vi "Tracks Button Adjust.vi"(0 "Left Forward Adjust":bool, 1 "Left Reverse Adjust":bool, 2 "Right Forward Adjust":bool, 3 "Right Reverse Adjust":bool, 4 "Adjust Speed":dbl, 5 "Drive 1":string="RobotDrive") -> ()   [LabVIEW 2017]
uses:
  <vilib>/Rock Robotics/WPI/Utilities/WPI_GetSetVariantRefNum.vi
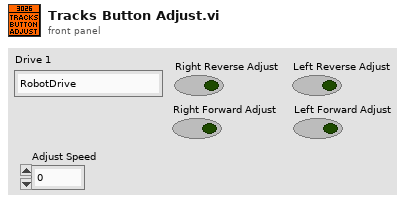
[diagram p1: front panel]
types:
  T1 = typedef "WPI_RobotDriveDevRef.ctl" = cluster{"DevStatus":errorcluster, "Motors[]":T2[], "Square Inputs":bool, "Max Output":dbl}
  T2 = typedef "WPI_MotorControlDeviceRef.ctl" = cluster{"DeviceStatus":errorcluster, "Type":T3, "PWM":cluster{"PWM Channel":T4, "DeadBand":T5}, "CAN":cluster{"Device Number":u8, "SetOutput VI Ref":variant, "GetOutput VI Ref":variant, "Enable VI Ref":variant, "Disable VI Ref":variant, "Data":variant}, "Invert":bool, "DIO PWM":cluster{"PWM \"Enable\" Channel":T4, "DIOChannel":T6, "PWM Rate":dbl}}
  T3 = typedef "WPI_MotorControlType.ctl" = enum16{"PWM", "CAN", "DIO PWM"}
  T4 = typedef "FPGA_DIOPWMChannel.ctl" = enum8{"PWM 0", "PWM 1", "PWM 2", "PWM 3", "PWM 4", "PWM 5", "PWM 6", "PWM 7", "PWM 8", "PWM 9", "PWM MXP 0", "PWM MXP 1", "PWM MXP 2", "PWM MXP 3", "PWM MXP 4", "PWM MXP 5", "PWM MXP 6", "PWM MXP 7", "PWM MXP 8", "PWM MXP 9", "Invalid"}
  T5 = typedef "WPI_PWMDeadband.ctl" = cluster{"Name":string, "maxPositivePwm":i32, "minPositivePwm":i32, "centerPwm":i32, "maxNegativePwm":i32, "minNegativePwm":i32, "angularRange":u16}
  T6 = typedef "FPGA_DIOChannel.ctl" = enum8{"DIO 0", "DIO 1", "DIO 2", "DIO 3", "DIO 4", "DIO 5", "DIO 6", "DIO 7", "DIO 8", "DIO 9", "DIO MXP 0", "DIO MXP 1", "DIO MXP 2", "DIO MXP 3", "DIO MXP 4", "DIO MXP 5", "DIO MXP 6", "DIO MXP 7", "DIO MXP 8", "DIO MXP 9", "DIO MXP 10", "DIO MXP 11", "DIO MXP 12", "DIO MXP 13", "DIO MXP 14", "DIO MXP 15", "SPI Port CS1", "SPI Port CS2", "SPI Port CS3", "SPI Port MISO", "SPI Port MOSI", "Invalid"}
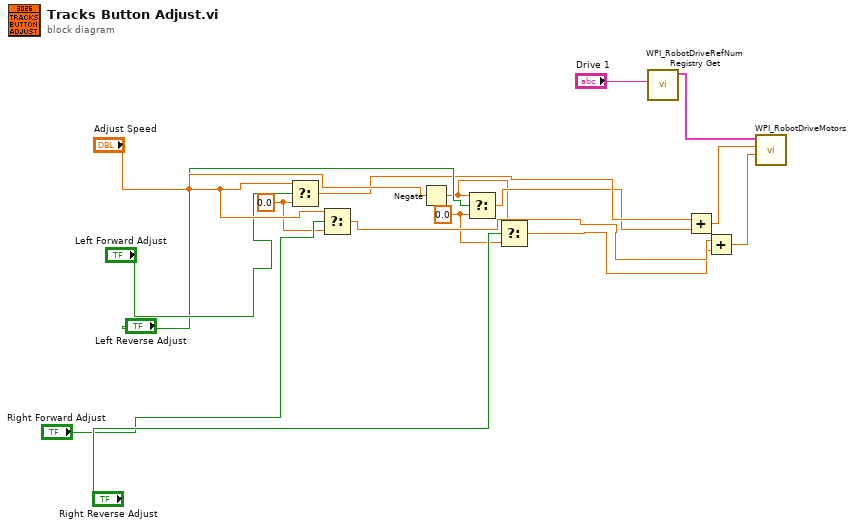
[diagram p0: block diagram]
diagram:
  w2 = 0.0 ("f")
  w1 = 0.0 ("f")
  n1 = Select(t="Adjust Speed", s="Left Forward Adjust", f=w1) -> (s? t:f=w9:dbl)
  n2 = Select(t="Adjust Speed", s="Right Forward Adjust", f=w1) -> (s? t:f=w7:dbl)
  n3 = Negate(x="Adjust Speed") -> (-x=w3:dbl)
  n4 = Select(t=w3, s="Left Reverse Adjust", f=w2) -> (s? t:f=w8:dbl)
  n5 = Select(t=w3, s="Right Reverse Adjust", f=w2) -> (s? t:f=w6:dbl)
  n6 = call <vilib>:"WPI_RobotDriveRefNum Registry Get.vi"("refnum name"="Drive 1") -> ("RobotDriveDevRef"=w16:T1)  [unwired: 9 in, 1 out]
  n7 = Add(x=w9, y=w8) -> (x+y=w4:dbl)
  n8 = Add(x=w7, y=w6) -> (x+y=w5:dbl)
  n9 = call <vilib>:"WPI_RobotDriveMotors.vi"("RightSpeed"=w5, "LeftSpeed"=w4, "RobotDriveDevRef"=w16) -> ()  [unwired: 6 in, 3 out]
